vi "simx_common.vi"() -> ()   [LabVIEW 2025]
doc: "This is a Global variable shared among all the sensors during the configuration phase. Contains the simx.ctl"
uses:
  controls/simx_connection.ctl
  controls/config.ctl
  controls/trajectory.ctl
  controls/weather.ctl
  controls/connections.ctl
  controls/start_points.ctl
  <vilib>/Utility/miscctls.llb/LVBoundsTypeDef.ctl
panel:
  in  "simx":T1={"Config"={"Trajectory"={"Number of frames"=0, "Frame number"=0, "Trajectory"=""}, "Weather"={"id"=""}}, "Connections"={"Simulator Connection"=refnum, "server_ip"="127.0.0.1", "Port"=0, "Sensor connections"=[]}, "Map"={"lanes"={"x"=[], "y"=[], "z"=[]}, "StartPosition"={"start_points"={"locations"=[], "rotations"=[], "type"=[]}, "StartRotation"=[], "StartLocation"=[]}, "Draw Map Size"={"Width"=800, "Height"=800}, "DrawArea"={"min_Y"=0.0, "min_X"=0.0, "Scale X"=0.0, "Scale Y"=0.0}, "Map"=bytes[0], "Map Geojson"=""}}
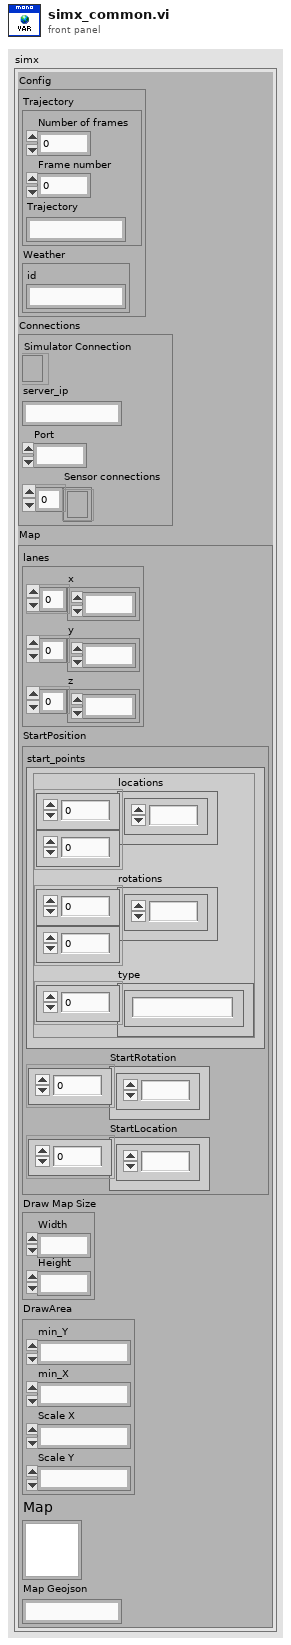
[diagram p1: front panel]
types:
  T1 = typedef "simx_connection.ctl" = cluster{"Config":T2, "Connections":T5, "Map":cluster{"lanes":cluster{"x":dbl[], "y":dbl[], "z":dbl[]}, "StartPosition":cluster{"start_points":T6, "StartRotation":dbl[], "StartLocation":dbl[]}, "Draw Map Size":T7, "DrawArea":cluster{"min_Y":dbl, "min_X":dbl, "Scale X":dbl, "Scale Y":dbl}, "Map":picture, "Map Geojson":string}}
  T2 = typedef "config.ctl" = cluster{"Trajectory":T3, "Weather":T4}
  T3 = typedef "trajectory.ctl" = cluster{"Number of frames":i32, "Frame number":i32, "Trajectory":string}
  T4 = typedef "weather.ctl" = cluster{"id":string}
  T5 = typedef "connections.ctl" = cluster{"Simulator Connection":refnum<k5>, "server_ip":string, "Port":i32, "Sensor connections":refnum<k5>[]}
  T6 = typedef "start_points.ctl" = cluster{"locations":dbl[][], "rotations":dbl[][], "type":string[]}
  T7 = typedef "LVBoundsTypeDef.ctl" = cluster{"Width":u32, "Height":u32}
diagram:
